vi "VFH Visualization.vi"() -> ()   [LabVIEW 2017]
uses:
  <vilib>/Platform/TimedLoop/XDataNode/timing_clust.ctl
  <vilib>/Platform/TimedLoop/XDataNode/nitl_modes.ctl
  <vilib>/Platform/TimedLoop/XDataNode/wakeup.ctl
  <vilib>/Analysis/coordinate.llb/Wrap Angle (scalar).vi
  <vilib>/Analysis/coordinate.llb/2D Cartesian Coordinate Rotation (Array).vi
  <vilib>/Platform/TimedLoop/XDataNode/XDataNode.xnode
  <vilib>/Platform/TimedLoop/XDataNode/XDNodeRunTimeDep.lvlib
  <vilib>/Analysis/NI_AALPro.lvlib
  <vilib>/Analysis/NI_AAL_Angle.lvlib
panel:
  out "VY History":dbl(graph)
  out "Heading History":dbl(graph)
  out "LIDAR data":cluster{dbl[], dbl[]}[](graph)
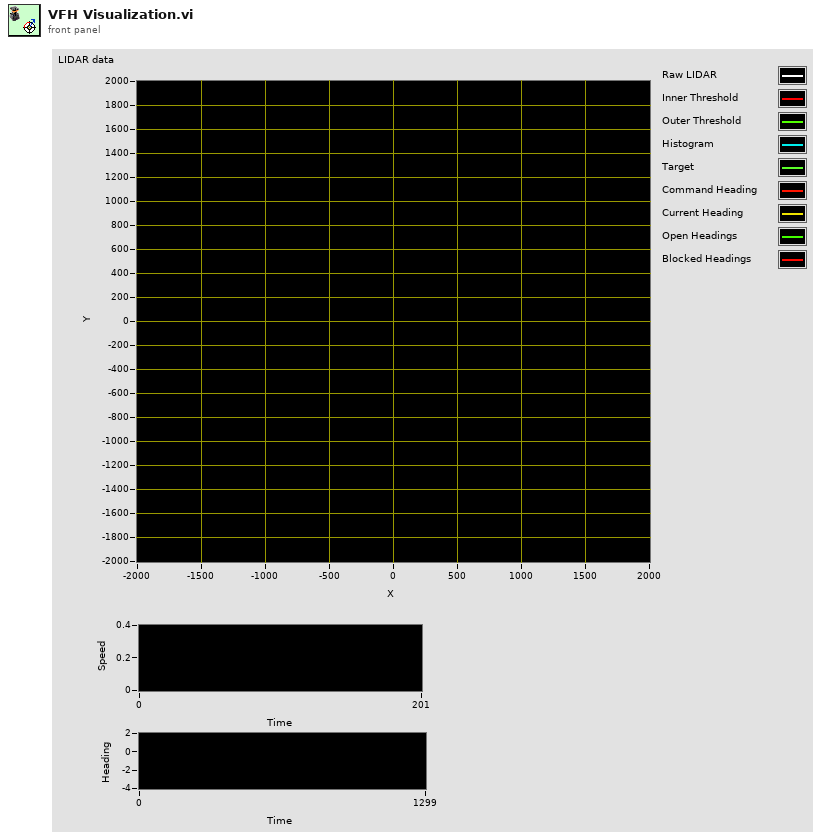
[diagram p1: front panel]
types:
  T1 = typedef "XDNodeRunTimeDep.lvlib/timing_clust.ctl" = cluster{"Expected End [f-1]":u64, "Actual End [f-1]":u64, "Finished Late? [f-1]":bool, "Expected End [i-1]":u64, "Actual End [i-1]":u64, "Finished Late? [i-1]":bool, "Expected Start [i]":u64, "Actual Start [i]":u64, "Expected Start [f]":u64, "Actual Start [f]":u64, "Source Name":string, "Structure Name":string, "Period":i64, "Deadline":i64, "Offset":i64, "Start":i64, "Priority":i32, "Timeout":i32, "Mode":T2, "Wakeup Reason":T3, "Error":errorcluster, "Source Type":string, "Secondary Source Type":string, "Global End Time":u64, "Global Start Time":u64, "Frame Duration":u64, "Iteration Duration":u64, "Assigned CPU":i32, "I/O Scan Engine Mode":u32}
  T2 = typedef "XDNodeRunTimeDep.lvlib/nitl_modes.ctl" = enum32{"No Change", "Process missed periods, maintain original phase", "Discard missed periods, maintain original phase", "Process missed periods, ignore original phase", "Discard missed periods, ignore original phase"}
  T3 = typedef "XDNodeRunTimeDep.lvlib/wakeup.ctl" = enum32{"Normal", "Aborted", "Asynchronous wakeup", "Timing source error", "Timed loop error", "Timeout"}
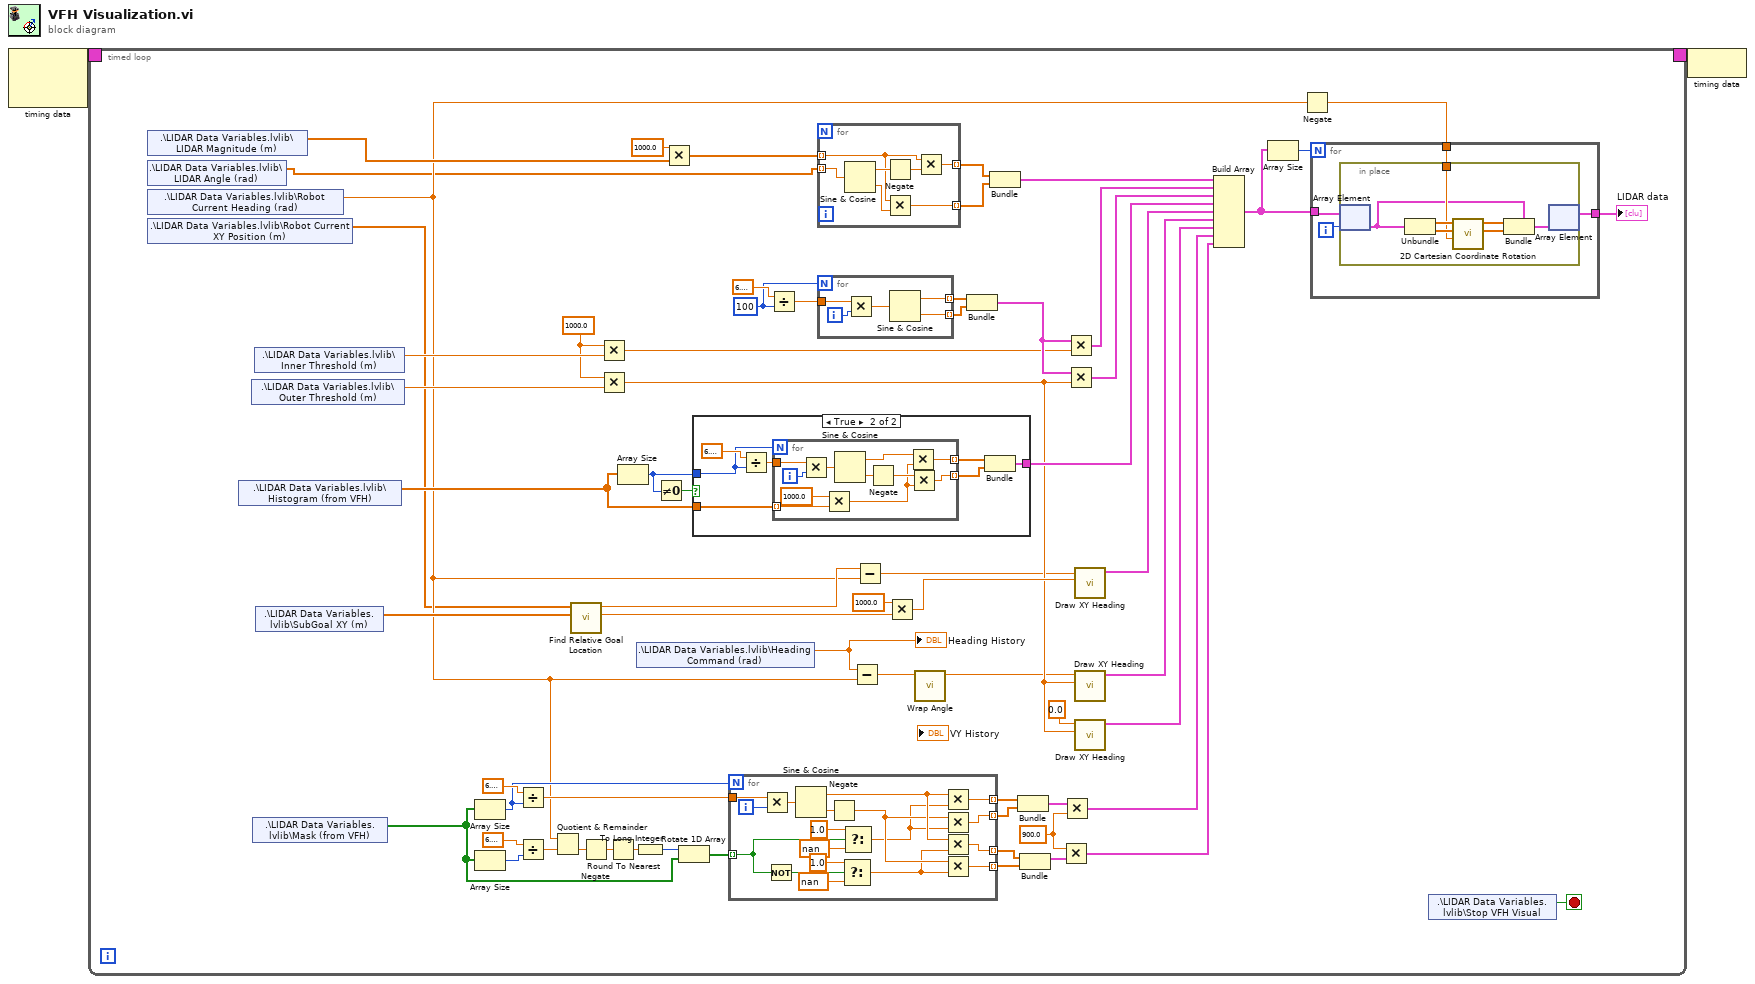
[diagram p0: block diagram]
diagram:
  n1 = node-c288() -> (w2:T1)  [unwired: 2 out]
  n2 = timed-loop {
    timing: w2 -> [_]
    timing-out: [_] -> w1
    stop <- w4 stop-if-true
    w18 = 1000.0 ("x")
    w10 = 900.0 ("y")
    w65 = 100 ("y")
    n3 = shared-variable ".\\LIDAR Data Variables.lvlib\\LIDAR Magnitude (m)"() -> (w7:dbl[])  [unwired: 1 in, 1 out]
    n4 = shared-variable ".\\LIDAR Data Variables.lvlib\\LIDAR Angle (rad)"() -> (w3:dbl[])  [unwired: 1 in, 1 out]
    n5 = shared-variable ".\\LIDAR Data Variables.lvlib\\Robot Current Heading (rad)"() -> (w6:dbl)  [unwired: 1 in, 1 out]
    n6 = shared-variable ".\\LIDAR Data Variables.lvlib\\Robot Current XY Position (m)"() -> (w5:dbl[])  [unwired: 1 in, 1 out]
    n7 = shared-variable ".\\LIDAR Data Variables.lvlib\\Histogram (from VFH)"() -> (w39:dbl[])  [unwired: 1 in, 1 out]
    n8 = shared-variable ".\\LIDAR Data Variables.lvlib\\Outer Threshold (m)"() -> (w22:dbl)  [unwired: 1 in, 1 out]
    n9 = shared-variable ".\\LIDAR Data Variables.lvlib\\Mask (from VFH)"() -> (w34:bool[])  [unwired: 1 in, 1 out]
    n10 = shared-variable ".\\LIDAR Data Variables.lvlib\\Inner Threshold (m)"() -> (w23:dbl)  [unwired: 1 in, 1 out]
    n11 = shared-variable ".\\LIDAR Data Variables.lvlib\\SubGoal XY (m)"() -> (w38:dbl[])  [unwired: 1 in, 1 out]
    n12 = Array Size(array=w34) -> (size(s)=w57:i32)
    n13 = Array Size(array=w34) -> (size(s)=w49:i32)
    n14 = Divide(x=6.283185307179586, y=w57) -> (x/y=w58:dbl)
    n15 = Divide(x=6.283185307179586, y=w49) -> (x/y=w48:dbl)
    n16 = Quotient & Remainder(x=w6, y=w48) -> (floor(x/y)=w47:dbl)  [unwired: 1 out]
    n17 = call "Find Relative Goal Location.vi"("Goal Position"=w38, "Current Position"=w5) -> ("Target Distance"=w35:dbl, "Target Heading"=w15:dbl)  [unwired: 8 in]
    n18 = Negate(x=w47) -> (-x=w46:dbl)
    n19 = Multiply(x=w18, y=w23) -> (x*y=w20:dbl)
    n20 = Multiply(x=w18, y=w22) -> (x*y=w19:dbl)
    n21 = Round To Nearest(number=w46) -> (nearest integer value=w45:dbl)
    n22 = Array Size(array=w39) -> (size(s)=w33:i32)
    n23 = To Long Integer(number=w45) -> (32bit integer=w44:i32)
    n24 = shared-variable ".\\LIDAR Data Variables.lvlib\\Heading Command (rad)"() -> (w25:dbl)  [unwired: 1 in, 1 out]
    "Heading History" <- w25
    n25 = Not Equal To 0?(x=w33) -> (x != 0?=w32:bool)
    n26 = Multiply(x=1000.0, y=w7) -> (x*y=w17:dbl[])
    n27 = Rotate 1D Array(1:w34, 2:w44) -> (0:w43:bool[])
    n28 = case shown="True" w32 {
      tunnel: [_ w74] -> w31
      tunnel: w39 -> [_ w69]
      tunnel: w33 -> [_ w68]
      frame False {
      }
      frame True {
        n29 = Divide(x=6.283185307179586, y=w68) -> (x/y=w71:dbl)
        n30 = for {
          N: w68 -> [_]
          tunnel: w71 -> [w84]
          tunnel: [w79] -> w72 mode=indexing
          tunnel: [w78] -> w73 mode=indexing
          tunnel: w69 -> [w77] mode=indexing
          i -> [w85]
          n31 = Multiply(x=w84, y=w85) -> (x*y=w83:dbl)
          n32 = Multiply(x=1000.0, y=w77) -> (x*y=w76:dbl)
          n33 = Sine & Cosine(0:w83) -> (1:w82:dbl, 2:w81:dbl)
          n34 = Negate(x=w81) -> (-x=w80:dbl)
          n35 = Multiply(x=w82, y=w76) -> (x*y=w79:dbl)
          n36 = Multiply(x=w80, y=w76) -> (x*y=w78:dbl)
        }
        n37 = Bundle(w72, w73) -> (w74:cluster{dbl[], dbl[]})  [unwired: 1 out]
      }
    }
    n38 = for {
      N: w57 -> [_]
      tunnel: w58 -> [w109]
      tunnel: [w100] -> w55 mode=indexing
      tunnel: [w99] -> w54 mode=indexing
      tunnel: w43 -> [w102] mode=indexing
      tunnel: [w97] -> w53 mode=indexing
      tunnel: [w98] -> w52 mode=indexing
      i -> [w110]
      n39 = Multiply(x=w109, y=w110) -> (x*y=w108:dbl)
      n40 = Not(x=w102) -> (.not. x?=w101:bool)
      n41 = Sine & Cosine(0:w108) -> (1:w96:dbl, 2:w107:dbl)
      n42 = Negate(x=w107) -> (-x=w95:dbl)
      n43 = Select(t=1.0, s=w101, f=nan) -> (s? t:f=w93:dbl)
      n44 = Select(t=1.0, s=w102, f=nan) -> (s? t:f=w94:dbl)
      n45 = Multiply(x=w96, y=w94) -> (x*y=w100:dbl)
      n46 = Multiply(x=w95, y=w94) -> (x*y=w99:dbl)
      n47 = Multiply(x=w96, y=w93) -> (x*y=w97:dbl)
      n48 = Multiply(x=w95, y=w93) -> (x*y=w98:dbl)
    }
    n49 = Divide(x=6.283185307179586, y=w65) -> (x/y=w64:dbl)
    n50 = for {
      tunnel: w17 -> [w86] mode=indexing
      tunnel: w3 -> [w87] mode=indexing
      tunnel: [w90] -> w40 mode=indexing
      tunnel: [w89] -> w41 mode=indexing
      n51 = Sine & Cosine(0:w87) -> (1:w92:dbl, 2:w91:dbl)
      n52 = Negate(x=w92) -> (-x=w88:dbl)
      n53 = Multiply(x=w86, y=w91) -> (x*y=w89:dbl)
      n54 = Multiply(x=w86, y=w88) -> (x*y=w90:dbl)
    }
    n55 = for {
      N: w65 -> [_]
      tunnel: w64 -> [w125]
      tunnel: [w123] -> w63 mode=indexing
      tunnel: [w122] -> w62 mode=indexing
      i -> [w126]
      n56 = Multiply(x=w125, y=w126) -> (x*y=w124:dbl)
      n57 = Sine & Cosine(0:w124) -> (1:w123:dbl, 2:w122:dbl)
    }
    n58 = Subtract(x=w25, y=w6) -> (x-y=w9:dbl)
    n59 = Subtract(x=w15, y=w6) -> (x-y=w14:dbl)
    n60 = Multiply(x=1000.0 ("y"), y=w35) -> (x*y=w36:dbl)
    n61 = call-poly <vilib>:"Wrap Angle.vi"("angle in"=w9) -> ("angle out"=w8:dbl)  [unwired: 9 in, 1 out]
    n62 = Bundle(w63, w62) -> (w21:cluster{dbl[], dbl[]})  [unwired: 1 out]
    n63 = Bundle(w40, w41) -> (w67:cluster{dbl[], dbl[]})  [unwired: 1 out]
    n64 = Bundle(w55, w54) -> (w56:cluster{dbl[], dbl[]})  [unwired: 1 out]
    n65 = Bundle(w53, w52) -> (w51:cluster{dbl[], dbl[]})  [unwired: 1 out]
    n66 = Multiply(x=w10, y=w51) -> (x*y=w26:cluster{dbl[], dbl[]})
    n67 = Multiply(x=w56, y=w10) -> (x*y=w27:cluster{dbl[], dbl[]})
    n68 = Multiply(x=w21, y=w20) -> (x*y=w24:cluster{dbl[], dbl[]})
    n69 = Multiply(x=w21, y=w19) -> (x*y=w61:cluster{dbl[], dbl[]})
    n70 = call "Draw XY Heading.vi"("Length"=w36, "Direction"=w14) -> ("Heading Graph"=w30:cluster{dbl[], dbl[]})  [unwired: 9 in]
    n71 = call "Draw XY Heading.vi"("Length"=w19, "Direction"=w8) -> ("Heading Graph"=w29:cluster{dbl[], dbl[]})  [unwired: 9 in]
    n72 = call "Draw XY Heading.vi"("Length"=w19, "Direction"=0.0) -> ("Heading Graph"=w28:cluster{dbl[], dbl[]})  [unwired: 9 in]
    n73 = Build Array(w67, w24, w61, w31, w30, w29, w28, w27, w26) -> (w12:cluster{dbl[], dbl[]}[])
    n74 = Array Size(array=w12) -> (size(s)=w11:i32)
    n75 = Negate(x=w6) -> (-x=w60:dbl)
    n76 = for {
      N: w11 -> [_]
      tunnel: w12 -> [w113]
      tunnel: w60 -> [w114]
      tunnel: [w112] -> w13
      i -> [w111]
      n77 = in-place {
        in-place-border: w114 -> [w117]
        n78 = in-place-array #1(w113, w111) -> (w116:cluster{dbl[], dbl[]})
        n79 = Unbundle(w116) -> (w121:dbl[], w120:dbl[])
        n80 = call-poly <vilib>:"2D Cartesian Coordinate Rotation.vi"("theta"=w117, "Y"=w120, "X"=w121) -> ("Y Out"=w118:dbl[], "X Out"=w119:dbl[])  [unwired: 6 in, 1 out]
        n81 = Bundle(cluster=w116, w119, w118) -> (w115:cluster{dbl[], dbl[]})
        n82 = in-place-array #1(w115) -> (w112:cluster{dbl[], dbl[]}[])  [unwired: 1 out]
      }
    }
    "LIDAR data" <- w13
    n83 = shared-variable ".\\LIDAR Data Variables.lvlib\\Stop VFH Visual"() -> (w4:bool)  [unwired: 1 in, 1 out]
  }
  n84 = node-c288(w1) -> ()
